vi "SaveConfigs_toFile.vi"(7 "ConfigFile Path":path=path "Default.conf.json", 11 "Configuration":T1={"Mode"="", "InstrumentMode"={"MainDAQ_Selector"=enum."None", "LaserCtrlMethod"=enum."SRS_DG535", "InstruMode"=enum."fsLDPI"}, "CommuniationSettings"={"SDG_II"="", "DG535"="", "BNC565"="", "EPM2000"="", "NI-DAQmx"="", "Micos"={"Simulation"=FALSE, "ComPort"="", "Serial Config"={"Baud Rate"=0, "Parity"=0, "Data Bits"=0, "Stop Bits"=0, "Flow Control"=0}, "#Axis"=0}, "ESP300"={"Simulation"=FALSE, "ComPort"="", "Serial Config"={"Baud Rate"=0, "Parity"=0, "Data Bits"=0, "Stop Bits"=0, "Flow Control"=0}, "#Axis"=0}}, "DG535"={"Trigger"={"Trigger Mode"=enum."Internal", "Internal/Burst Rate"=0.0, "External  Level"=0.0, "Impedance"=FALSE, "Slope"=FALSE}, "Delays"=[], "Output"=[]}, "Gage_Config"={"Acquisition"={"Sample Rate"=0.0, "Mode"=0, "Start (0)"=0.0, "Depth"=0.0, "Segment Size"=0.0, "Trigger Delay"=0.0, "Trigger Timeout"=0.0, "Trigger Holdoff"=0.0, "Clock mode"=enum."Internal", "Segment"=1}, "Channels"=[], "Trigger"={"Slope"=0, "Level"=0, "Source"=0, "External Range"=0, "External Coupling"=0, "External"=FALSE, "Disable"=FALSE, "External Impedance"=0}, "Mode(Gage)"=enum."Normal"}, "AnalogDisc_Config"={"Acqusition"={"Freq(Hz,SampleRate)"=0.0, "BufferSize"=0, "Mode"=enum."Single", "RecordLength(s)"=0.0}, "Channels"=[], "Trigger"={"TriggerSource"=enum."None", "Timeout(s)"=0.0, "Holdoff(s)"=0.0, "Position/Delay(s)"=0.0}, "AnalogTrigger"={"Channel"=0, "Polarity"=enum."Rising", "Type"=enum."Edge", "Level(V)"=0.0, "Filter"=enum."Decimate", "Hysterisis(V)"=0.0}}, "Micos"={"Velocity"=0.0, "Acceleration"=0.0}, "ESP300"={"Velocity"=[], "Acceleration"=[]}, "EPM2000"={"Factor(A)"=0.0, "Factor(B)"=0.0}, "ProcessMethod"={"TopLine"=0.0, "Threshold"=0.0, "Baseline"=0.0, "ZeroOffset"=0.0, "Processing Mode"=enum."None"}, "Timing(LDPI)"={"Delay(PI)"=0.0, "Delay(Rejection)"=0.0, "NoDelayOffset"=0.0, "RepRate(Hz)"=0.0}, "Cali."=[0.0707, 0.16163, 0.02539], "BNC_Config"={"System"={"Rep.Rate"=1000.0, "Sys Ext Mode"=enum."Triggered", "Mode"=enum."Single Shot"}, "Channels"=[]}} {"Cali." format="%#.6f"; "Timing(LDPI)"."Delay(PI)" format="%#_6p"; "Timing(LDPI)"."Delay(Rejection)" format="%#_6p"; "Timing(LDPI)"."NoDelayOffset" format="%#_6p"; "DG535"."Trigger"."External  Level" min=-2.56 max=2.56 format="%.2f"; "DG535"."Trigger"."Internal/Burst Rate" min=0.001 max=1000000.0 format="%.3f"; "DG535"."Delays"."Delay" format="%#_6p"; "DG535"."Output"."Offset" min=-3.0 max=4.0 format="%.2f"; "DG535"."Output"."Amplitude" min=-3.0 max=4.0 format="%.2f"; "ProcessMethod"."Threshold" format="%#_6p"; "Gage_Config"."Trigger"."External Impedance" items=["50 Ohm", "HiZ"]; "Gage_Config"."Trigger"."External Coupling" items=["DC", "AC"]; "Gage_Config"."Trigger"."External Range" min=2000 max=10000 step=8000; "Gage_Config"."Trigger"."Slope" items=["Rising", "Falling"]; "Gage_Config"."Trigger"."Level" min=-100 max=100; "Gage_Config"."Trigger"."Source" min=0 max=64 step=1; "Gage_Config"."Channels"."Impedance" min=50 max=1000000 step=999950; "Gage_Config"."Channels"."Coupling" items=["DC", "AC"]; "Gage_Config"."Acquisition"."Segment Size" min=256.0 step=128.0; "Gage_Config"."Acquisition"."Trigger Delay" min=0.0 step=128.0; "Gage_Config"."Acquisition"."Trigger Timeout" format="%.0p"; "Gage_Config"."Acquisition"."Trigger Holdoff" min=0.0 step=128.0; "Gage_Config"."Acquisition"."Depth" min=256.0 step=128.0; "Gage_Config"."Acquisition"."Mode" items=["Single", "Dual", "Quad", "Octal"]; "Gage_Config"."Acquisition"."Sample Rate" format="%.0p"; "AnalogDisc_Config"."AnalogTrigger"."Level(V)" format="%#_6p"; "AnalogDisc_Config"."AnalogTrigger"."Hysterisis(V)" format="%#_6p"; "AnalogDisc_Config"."Acqusition"."RecordLength(s)" format="%#_6p"; "AnalogDisc_Config"."Acqusition"."Freq(Hz,SampleRate)" format="%#_6p"; "AnalogDisc_Config"."Trigger"."Position/Delay(s)" format="%#_6p"; "AnalogDisc_Config"."Trigger"."Holdoff(s)" format="%#_6p"; "AnalogDisc_Config"."Trigger"."Timeout(s)" format="%#_6p"}) -> ()   [LabVIEW 2013]
uses:
  ControlDef/InstrumentConfiguration.ctl
  ControlDef/MainDAQ_Selector.ctl
  ControlDef/LaserCtrl_Method.ctl
  ControlDef/InstruMode_Typedef.ctl
  <instrlib>/DG535/Command/Set Trigger.ctl
  <instrlib>/DG535/Command/DG535_TriggerMode.ctl
  <instrlib>/DG535/Command/Set Delay.ctl
  <instrlib>/DG535/Command/DG535_Channel.ctl
  <instrlib>/DG535/Command/Set Output.ctl
  <instrlib>/DG535/Command/DG535_Output.ctl
  <instrlib>/GageLv_uic/VI/Gage_Configs.ctl
  <instrlib>/AnalogDiscSDKLv/VIs/DWF_AnalogIn_Configurations.ctl
  <instrlib>/AnalogDiscSDKLv/VIs/DWF_AcqMode.ctl
  <instrlib>/AnalogDiscSDKLv/VIs/DWF_Filter.ctl
  <instrlib>/AnalogDiscSDKLv/VIs/DWF_TrigSrc.ctl
  <instrlib>/AnalogDiscSDKLv/VIs/DWF_TrigCond.ctl
  <instrlib>/AnalogDiscSDKLv/VIs/DWF_TrigType.ctl
  ControlDef/ProcessingMode.ctl
  Hardware/BNC(QuantumComposers)/BNC_Configs.ctl
  ControlDef/InstrumentSpecificControls/UIC-AToF/InitializationParams_BNC565_2Ch_AToF.ctl
  Hardware/BNC(QuantumComposers)/Command/Set C-Input.ctl
  Hardware/BNC(QuantumComposers)/Command/Set C-Mode.ctl
  Hardware/BNC(QuantumComposers)/Command/Set C-Output.ctl
  Hardware/BNC(QuantumComposers)/Command/Set C-Enable.ctl
  <vilib>/addons/JSON API/JSON Value/JSON Value.lvclass
  <vilib>/addons/JSON API/Variant JSON/Variant JSON.lvlib
  <instrlib>/AnalogDiscSDKLv/AnalogDiscSDKLv.lvlib
  <instrlib>/GageLv_uic/Gage.lvlib
  <instrlib>/DG535/SRS_DG535_Lib.lvlib
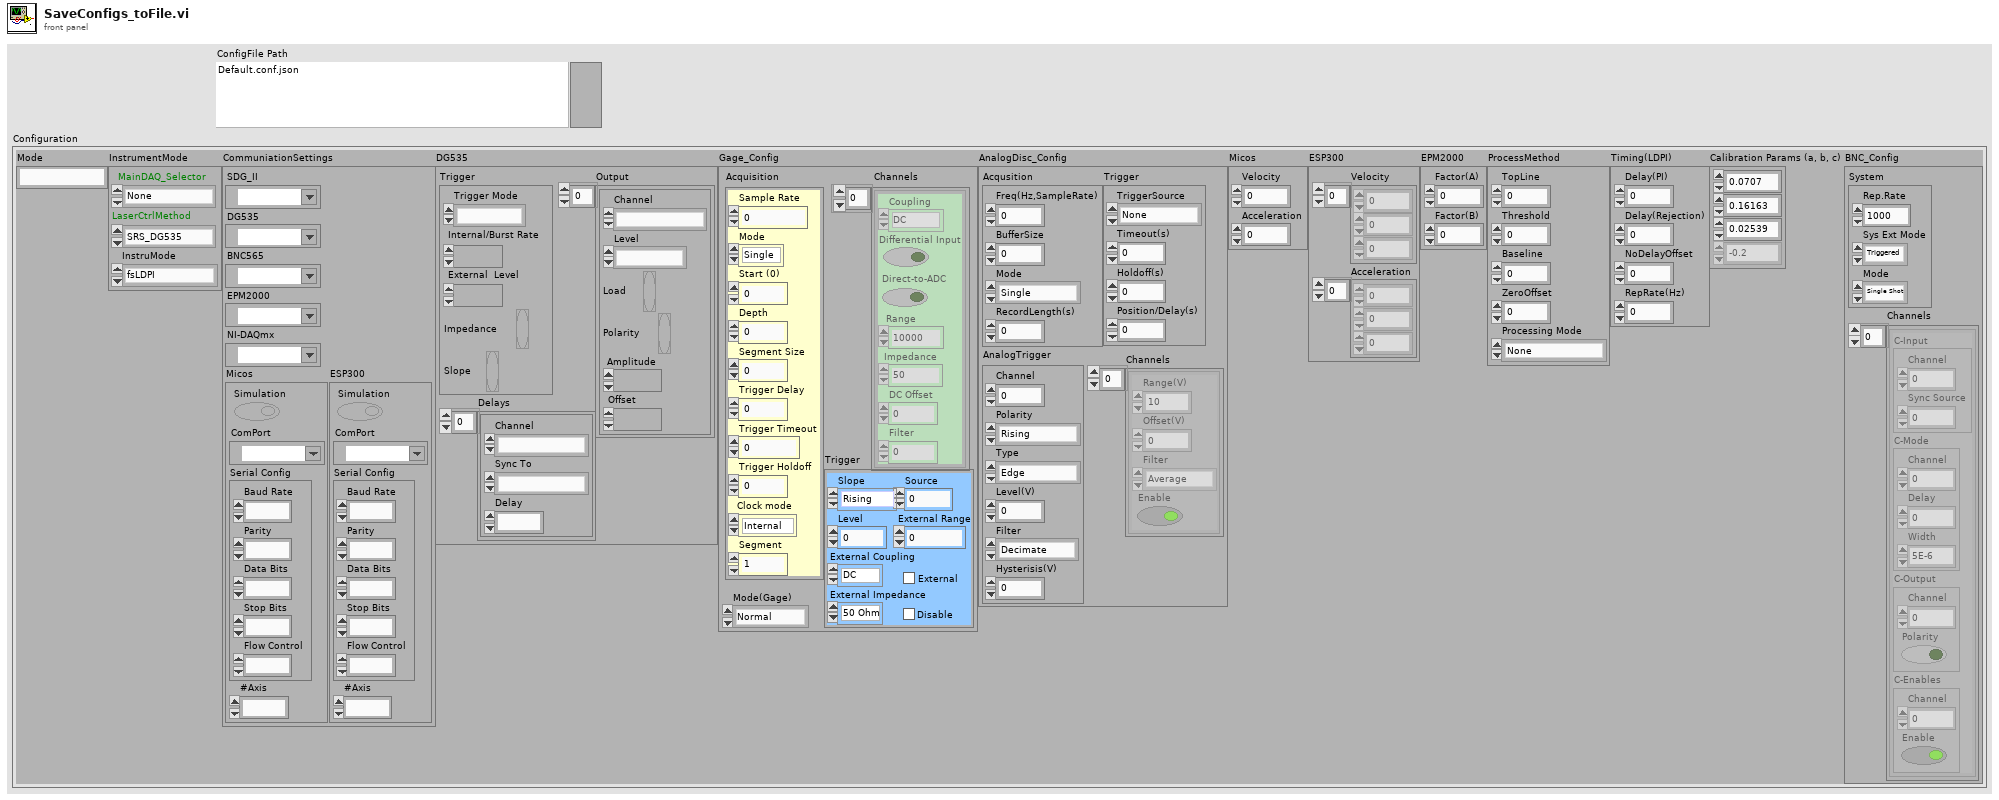
[diagram p1: front panel]
types:
  T1 = typedef "InstrumentConfiguration.ctl" = cluster{"Mode":string, "InstrumentMode":cluster{"MainDAQ_Selector":T2, "LaserCtrlMethod":T3, "InstruMode":T4}, "CommuniationSettings":cluster{"SDG_II":refnum<visa-resource-name>, "DG535":refnum<visa-resource-name>, "BNC565":refnum<visa-resource-name>, "EPM2000":refnum<visa-resource-name>, "NI-DAQmx":refnum<visa-resource-name>, "Micos":cluster{"Simulation":bool, "ComPort":refnum<visa-resource-name>, "Serial Config":cluster{"Baud Rate":u32, "Parity":u16, "Data Bits":u16, "Stop Bits":u16, "Flow Control":u16}, "#Axis":i32}, "ESP300":cluster{"Simulation":bool, "ComPort":refnum<visa-resource-name>, "Serial Config":cluster{"Baud Rate":u32, "Parity":u16, "Data Bits":u16, "Stop Bits":u16, "Flow Control":u16}, "#Axis":i32}}, "DG535":cluster{"Trigger":T5, "Delays":T7[], "Output":T9[]}, "Gage_Config":T11, "AnalogDisc_Config":T12, "Micos":cluster{"Velocity":dbl, "Acceleration":dbl}, "ESP300":cluster{"Velocity":dbl[], "Acceleration":dbl[]}, "EPM2000":cluster{"Factor(A)":dbl, "Factor(B)":dbl}, "ProcessMethod":cluster{"TopLine":dbl, "Threshold":dbl, "Baseline":dbl, "ZeroOffset":dbl, "Processing Mode":T18}, "Timing(LDPI)":cluster{"Delay(PI)":dbl, "Delay(Rejection)":dbl, "NoDelayOffset":dbl, "RepRate(Hz)":dbl}, "Cali.":dbl[], "BNC_Config":T19}
  T2 = typedef "MainDAQ_Selector.ctl" = enum16{"None", "Gage", "Gage_AdvMultiRec_8bit1Ch", "IonWerks_TDCx4", "Tektronics", "KnifeEdge_Emu", "AnalogDisc", "Gage_AMR_8bit2Ch", "Gage_AMR_16bit1Ch", "Gage_AMR_16bit2Ch", "FakeSignal(Emulator)"}
  T3 = typedef "LaserCtrl_Method.ctl" = enum16{"SRS_DG535", "BNC", "SDG_II"}
  T4 = typedef "InstruMode_Typedef.ctl" = enum16{"fsLDPI", "nsLDPI", "nsLD-fsPI", "GenericTOF", "BeamProfiling"}
  T5 = typedef "SRS_DG535_Lib.lvlib/Set Trigger.ctl" = cluster{"Trigger Mode":T6, "Internal/Burst Rate":dbl, "External  Level":sgl, "Impedance":bool, "Slope":bool}
  T6 = typedef "SRS_DG535_Lib.lvlib/DG535_TriggerMode.ctl" = enum16{"Internal", "External", "SingleShot", "Burst", "Line"}
  T7 = typedef "SRS_DG535_Lib.lvlib/Set Delay.ctl" = cluster{"Channel":T8, "Sync To":T8, "Delay":dbl}
  T8 = typedef "SRS_DG535_Lib.lvlib/DG535_Channel.ctl" = enum16{"Trigger Input", "T0 Output", "A Output", "B Output", "AB Output", "C Output", "D Output", "CD Output", "NULL"}
  T9 = typedef "SRS_DG535_Lib.lvlib/Set Output.ctl" = cluster{"Channel":T8, "Level":T10, "Load":bool, "Polarity":bool, "Amplitude":dbl, "Offset":dbl}
  T10 = typedef "SRS_DG535_Lib.lvlib/DG535_Output.ctl" = enum16{"TTL", "NIM", "ECL", "Variable"}
  T11 = typedef "Gage.lvlib/Gage_Configs.ctl" = cluster{"Acquisition":cluster{"Sample Rate":dbl, "Mode":u16, "Start (0)":dbl, "Depth":dbl, "Segment Size":dbl, "Trigger Delay":dbl, "Trigger Timeout":dbl, "Trigger Holdoff":dbl, "Clock mode":enum16{"Internal", "External", "Reference"}, "Segment":u32}, "Channels":cluster{"Coupling":u16, "Differential Input":bool, "Direct-to-ADC":bool, "Range":u32, "Impedance":u32, "DC Offset":i32, "Filter":i32}[], "Trigger":cluster{"Slope":u16, "Level":i32, "Source":i32, "External Range":u32, "External Coupling":u16, "External":bool, "Disable":bool, "External Impedance":u16}, "Mode(Gage)":enum16{"Normal", "Continuous", "MultiRecord", "HwAverage"}}
  T12 = typedef "AnalogDiscSDKLv.lvlib/DWF_AnalogIn_Configurations.ctl" = cluster{"Acqusition":cluster{"Freq(Hz,SampleRate)":dbl, "BufferSize":i32, "Mode":T13, "RecordLength(s)":dbl}, "Channels":cluster{"Range(V)":dbl, "Offset(V)":dbl, "Filter":T14, "Enable":bool}[], "Trigger":cluster{"TriggerSource":T15, "Timeout(s)":dbl, "Holdoff(s)":dbl, "Position/Delay(s)":dbl}, "AnalogTrigger":cluster{"Channel":i32, "Polarity":T16, "Type":T17, "Level(V)":dbl, "Filter":T14, "Hysterisis(V)":dbl}}
  T13 = typedef "AnalogDiscSDKLv.lvlib/DWF_AcqMode.ctl" = enum16{"Single", "ScanShift", "ScanScreen", "Record"}
  T14 = typedef "AnalogDiscSDKLv.lvlib/DWF_Filter.ctl" = enum16{"Decimate", "Average", "MinMax"}
  T15 = typedef "AnalogDiscSDKLv.lvlib/DWF_TrigSrc.ctl" = enum16{"None", "PC", "DetectorAnalogIn", "DetectorDigitalIn", "AnalogIn", "DigitalIn", "DigitalOut", "AnalogOut1", "AnalogOut2", "AnalogOut3", "AnalogOut4", "External1", "External2", "External3", "External4"}
  T16 = typedef "AnalogDiscSDKLv.lvlib/DWF_TrigCond.ctl" = enum16{"Rising", "Falling"}
  T17 = typedef "AnalogDiscSDKLv.lvlib/DWF_TrigType.ctl" = enum16{"Edge", "Pulse", "Transition"}
  T18 = typedef "ProcessingMode.ctl" = enum16{"None", "Drop by Threshold", "TDC Simulate", "SetFilter"}
  T19 = typedef "BNC_Configs.ctl" = cluster{"System":cluster{"Rep.Rate":dbl, "Sys Ext Mode":enum16{"Disabled", "Triggered", "Gated", "Triggered & Gated"}, "Mode":enum16{"Normal", "Single Shot", "Duty Cycle", "Burst"}}, "Channels":T20[]}
  T20 = typedef "InitializationParams_BNC565_2Ch_AToF.ctl" = cluster{"C-Input":T21, "C-Mode":T22, "C-Output":T23, "C-Enables":T24}
  T21 = typedef "Set C-Input.ctl" = cluster{"Channel":i32, "Sync Source":i32}
  T22 = typedef "Set C-Mode.ctl" = cluster{"Channel":i32, "Delay":dbl, "Width":dbl}
  T23 = typedef "Set C-Output.ctl" = cluster{"Channel":i32, "Polarity":bool}
  T24 = typedef "Set C-Enable.ctl" = cluster{"Channel":i32, "Enable":bool}
  T25 = enum16{"open", "replace", "create", "open or create", "replace or create", "replace or create with confirmation"}
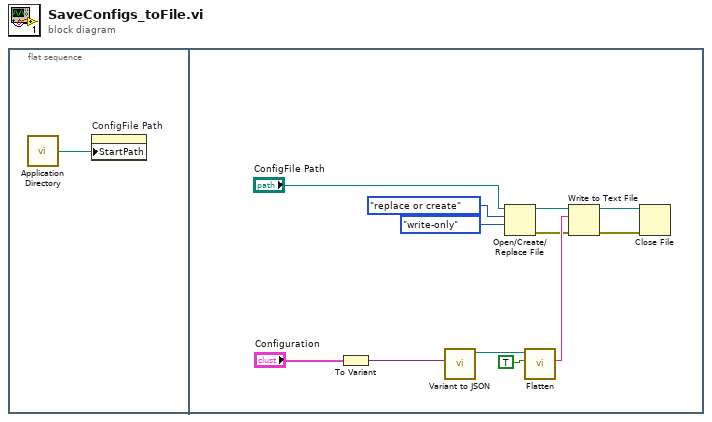
[diagram p0: block diagram]
diagram:
  n1 = flat-sequence {
    frame #0 {
      n2 = call <vilib>:"Application Directory.vi"() -> ("Application Directory"=w1:path)
      n3 = property on="ConfigFile Path" class="Path"("StartPath"=w1) -> ()  [unwired: 2 in, 2 out]
    }
    frame #1 {
      n4 = To Variant(anything="Configuration") -> (Variant=w6:variant)
      n5 = call <vilib>:"Variant to JSON.vi"("Variant"=w6) -> ("JSON Value out"=w13:refnum<class "JSON Value.lvclass">)  [unwired: 9 in, 1 out]
      n6 = Open/Create/Replace File(file path (use dialog)="ConfigFile Path", operation (0:open)=T25."replace or create", access (0:read/write)=enum16{"read/write", "read-only", "write-only"}."write-only") -> (refnum out=w11:refnum<file>, error out=w5:errorcluster)  [unwired: 3 in, 1 out]
      n7 = call-dynamic "Flatten.vi"("Pretty Print?"=TRUE, "JSON Value in"=w13) -> ("String"=w7:string)  [unwired: 8 in, 1 out]
      n8 = Write to Text File(file (use dialog)=w11, text=w7, error in=w5) -> (refnum out=w8:refnum<file>, error out=w4:errorcluster)  [unwired: 1 in, 1 out]
      n9 = Close File(refnum=w8, error in=w4) -> ()  [unwired: 2 out]
    }
  }
